vi "Microstrain IMU.vi"() -> ()   [LabVIEW 2012]
uses:
  <instrlib>/MicroStrain 3DM-GX1/MicroStrain 3DM-GX1.lvlib
  <vilib>/Platform/TimedLoop/XDataNode/wakeup.ctl
  <vilib>/Platform/TimedLoop/XDataNode/XDNodeRunTimeDep.lvlib
  <vilib>/Platform/TimedLoop/XDataNode/nitl_modes.ctl
  <vilib>/Platform/TimedLoop/XDataNode/timing_clust.ctl
  <vilib>/Platform/TimedLoop/XDataNode/XDataNode.xnode
  <vilib>/robotics/Controls/Compass Indicator/Compass Indicator.xctl
panel:
  out "VI Name":string
  out "Angle":dbl
  out "Waveform Chart 2":T1(graph)
  out "Waveform Chart":cluster{"Roll":dbl, "Pitch":dbl, "Yaw":dbl}(graph)
  in  "stop?":bool
  out "IMU Data":T2 {"Quaternion" format="%#.4g"; "Angular Rate"."Z-Axis Angular Rate" format="%#.4g"; "Angular Rate"."Y-Axis Angular Rate" format="%#.4g"; "Angular Rate"."X-Axis Angular Rate" format="%#.4g"; "Acceleration"."X-Axis Acceleration" format="%#.4g"; "Acceleration"."Y-Axis Acceleration" format="%#.4g"; "Acceleration"."Z-Axis Acceleration" format="%#.4g"; "Magnetic Field"."X-Axis Magnetic Field" format="%#.4g"; "Magnetic Field"."Y-Axis Magnetic Field" format="%#.4g"; "Magnetic Field"."Z-Axis Magnetic Field" format="%#.4g"; "Orientation Matrix" format="%#.4g"; "Position"."Yaw" format="%#.2f"; "Position"."Pitch" format="%#.1f"; "Position"."Roll" format="%#.1f"}
  in  "North Offset":dbl=30.0
  out "Compass Indicator":dbl(xcontrol)
  out "error out":errorcluster
  in  "Baud Rate":u32(ring)=115200 items=["19200"=19200, "38400"=38400, "115200"=115200]
  in  "Debug":bool
  in  "VISA resource name":refnum<visa-resource-name>="COM13"
  in  "Configure":bool
  out "Error Display":errorcluster
  in  "Enable Gyro-Stabilization (Enable)":bool=TRUE
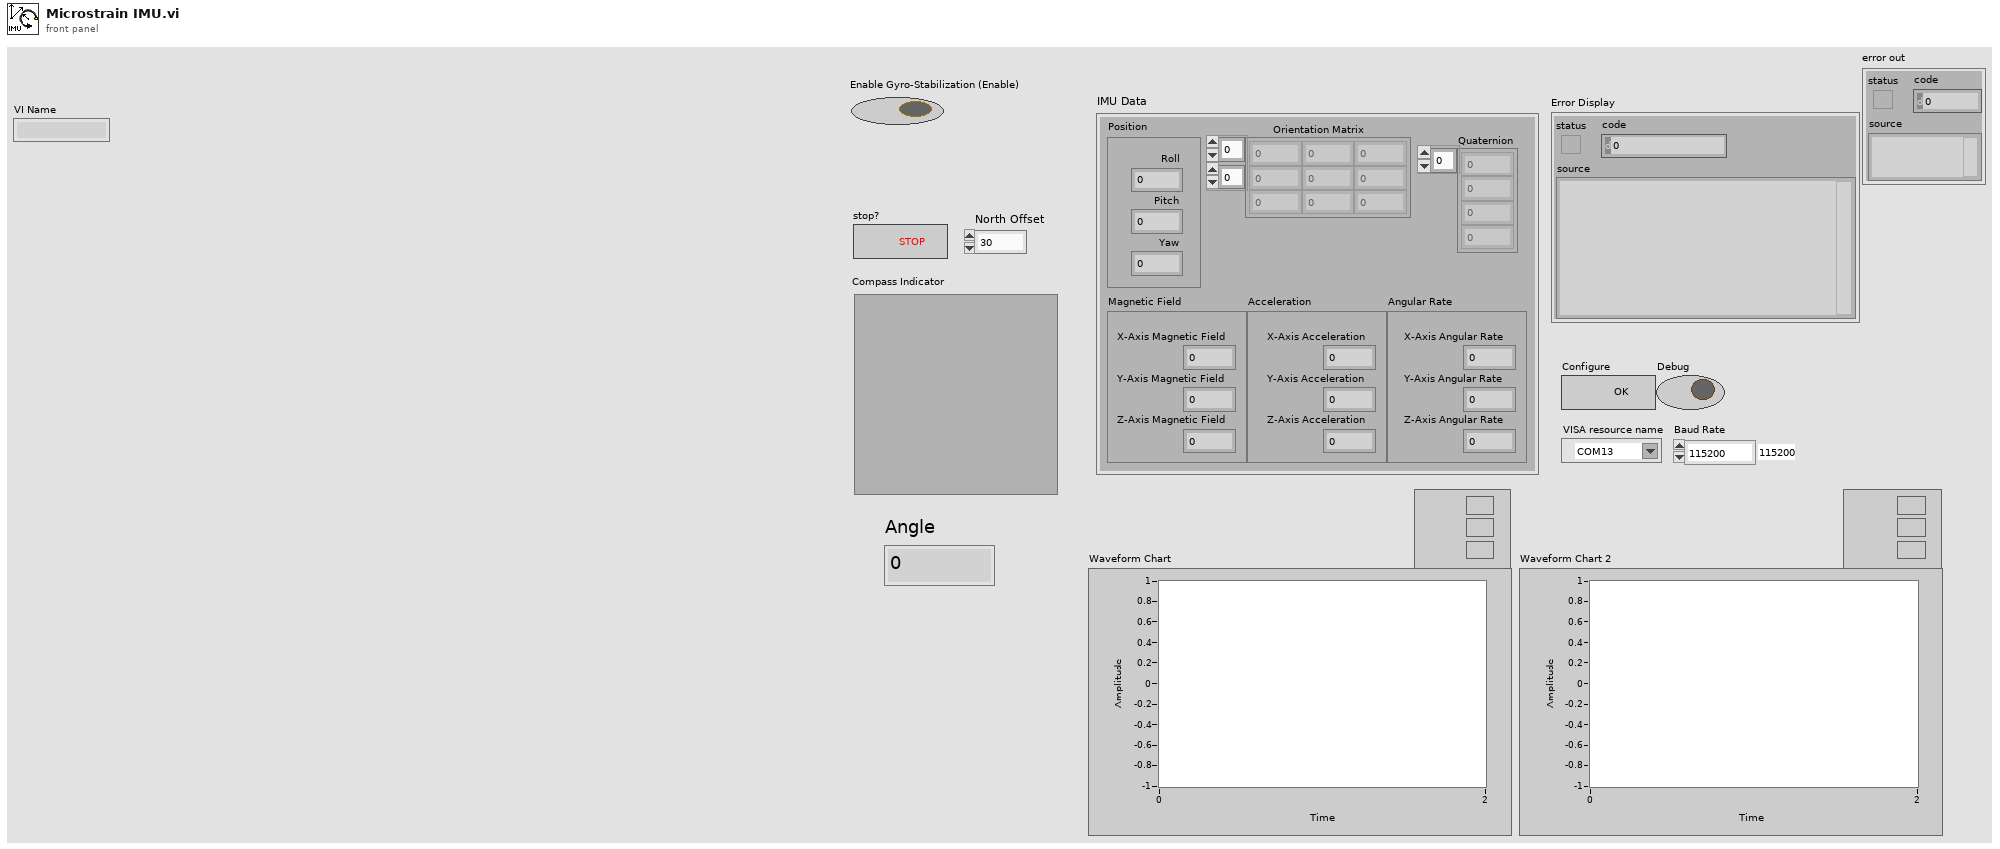
[diagram p1: front panel]
types:
  T1 = cluster{"X-Axis Magnetic Field":dbl, "Y-Axis Magnetic Field":dbl, "Z-Axis Magnetic Field":dbl}
  T2 = cluster{"Position":cluster{"Roll":dbl, "Pitch":dbl, "Yaw":dbl}, "Orientation Matrix":dbl[][], "Magnetic Field":cluster{"Z-Axis Magnetic Field":dbl, "Y-Axis Magnetic Field":dbl, "X-Axis Magnetic Field":dbl}, "Acceleration":cluster{"Z-Axis Acceleration":dbl, "Y-Axis Acceleration":dbl, "X-Axis Acceleration":dbl}, "Angular Rate":cluster{"X-Axis Angular Rate":dbl, "Y-Axis Angular Rate":dbl, "Z-Axis Angular Rate":dbl}, "Quaternion":dbl[]}
  T3 = typedef "XDNodeRunTimeDep.lvlib/timing_clust.ctl" = cluster{"Expected End [f-1]":u64, "Actual End [f-1]":u64, "Finished Late? [f-1]":bool, "Expected End [i-1]":u64, "Actual End [i-1]":u64, "Finished Late? [i-1]":bool, "Expected Start [i]":u64, "Actual Start [i]":u64, "Expected Start [f]":u64, "Actual Start [f]":u64, "Source Name":string, "Structure Name":string, "Period":i64, "Deadline":i64, "Offset":i64, "Start":i64, "Priority":i32, "Timeout":i32, "Mode":T4, "Wakeup Reason":T5, "Error":errorcluster, "Source Type":string, "Secondary Source Type":string, "Global End Time":u64, "Global Start Time":u64, "Frame Duration":u64, "Iteration Duration":u64, "Assigned CPU":i32, "I/O Scan Engine Mode":u32}
  T4 = typedef "XDNodeRunTimeDep.lvlib/nitl_modes.ctl" = enum32{"No Change", "Process missed periods, maintain original phase", "Discard missed periods, maintain original phase", "Process missed periods, ignore original phase", "Discard missed periods, ignore original phase"}
  T5 = typedef "XDNodeRunTimeDep.lvlib/wakeup.ctl" = enum32{"Normal", "Aborted", "Asynchronous wakeup", "Timing source error", "Timed loop error", "Timeout"}
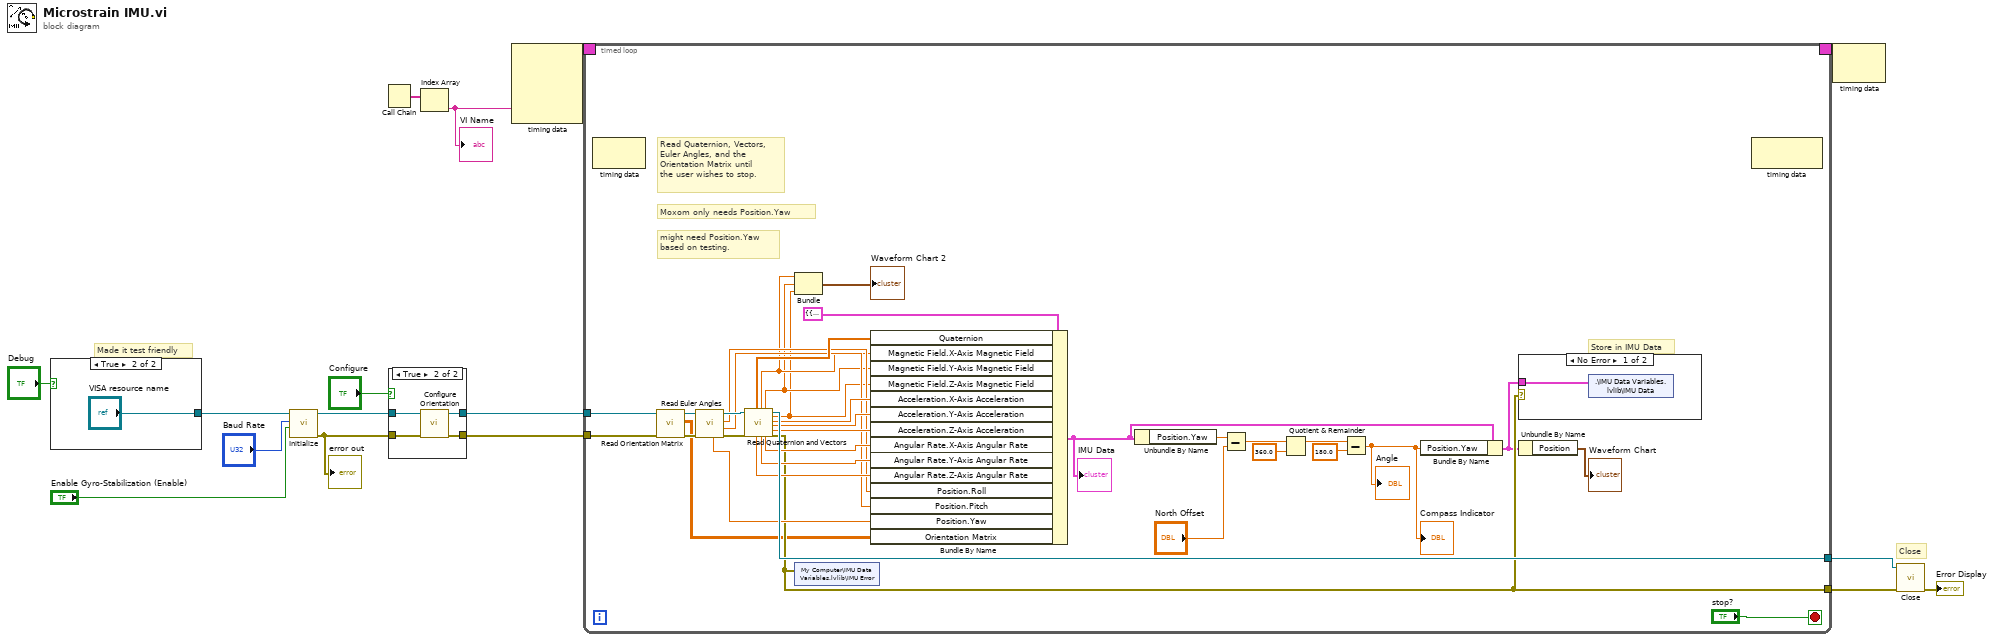
[diagram p0: block diagram]
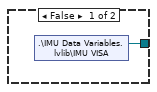
[diagram p3: hidden frame]
diagram:
  # "Made it test friendly"
  # "Close"
  n1 = case shown="True" "Debug" {
    tunnel: [w17 "VISA resource name"] -> w9
    frame False {
      n2 = shared-variable ".\\IMU Data Variables.lvlib\\IMU VISA"() -> (w17:refnum<visa-resource-name>)  [unwired: 1 in, 1 out]
    }
    frame True {
    }
  }
  n3 = call <instrlib>:"Initialize.vi"("Enable Gyro-Stabilization (True)"="Enable Gyro-Stabilization (Enable)", "Baud Rate (38400)"="Baud Rate", "VISA resource name"=w9) -> ("error out"=w13:errorcluster, "VISA resource name out"=w14:refnum<visa-resource-name>)  [unwired: 7 in]
  "error out" <- w13
  n4 = Call Chain() -> (call chain=w2:string[])
  n5 = case shown="True" "Configure" {
    tunnel: w14 -> [w20 w24]
    tunnel: w13 -> [w19 w23]
    tunnel: [w20 w22] -> w4
    tunnel: [w19 w21] -> w3
    frame False {
    }
    frame True {
      n6 = call <instrlib>:"Configure Orientation.vi"("error in (no error)"=w23, "VISA resource name"=w24) -> ("error out"=w21:errorcluster, "VISA resource name out"=w22:refnum<visa-resource-name>)  [unwired: 8 in]
    }
  }
  n7 = Index Array(array=w2) -> (element=w1:string)  [unwired: 1 in]
  "VI Name" <- w1
  n8 = node-c288(w1) -> (w16:T3)  [unwired: 3 in]
  n9 = timed-loop {
    tunnel: [w43] -> w12
    tunnel: [w57] -> w11
    timing: w16 -> [_]
    timing-out: [_] -> w15
    tunnel: w4 -> [w38]
    tunnel: w3 -> [w37]
    stop <- "stop?" stop-if-true
    # "Moxom only needs Position.Yaw"
    # "Store in IMU Data"
    # "might need Position.Yaw\nbased on testing."
    # "Read Quaternion, Vectors,\nEuler Angles, and the\nOrientation Matrix until\nthe user wishes to stop."
    n10 = node-c288() -> ()  [unwired: 1 in, 1 out]
    n11 = call <instrlib>:"Read Orientation Matrix.vi"("error in (no error)"=w37, "VISA resource name"=w38) -> ("error out"=w58:errorcluster, "Orientation Matrix"=w42:dbl[][], "VISA resource name out"=w59:refnum<visa-resource-name>)  [unwired: 7 in]
    n12 = call <instrlib>:"Read Euler Angles.vi"("error in (no error)"=w58, "VISA resource name"=w59) -> ("error out"=w55:errorcluster, "Pitch"=w44:dbl, "Roll"=w46:dbl, "VISA resource name out"=w56:refnum<visa-resource-name>, "Yaw"=w45:dbl)  [unwired: 5 in]
    n13 = call <instrlib>:"Read Quaternion and Vectors.vi"("VISA resource name"=w56, "error in (no error)"=w55) -> ("Quaternion"=w53:dbl[], "Z-Axis Angular Rate"=w47:dbl, "X-Axis Magnetic Field"=w36:dbl, "Y-Axis Angular Rate"=w48:dbl, "Y-Axis Magnetic Field"=w35:dbl, "X-Axis Angular Rate"=w49:dbl, "VISA resource name out"=w57:refnum<visa-resource-name>, "Z-Axis Magnetic Field"=w34:dbl, "X-Axis Acceleration"=w52:dbl, "Y-Axis Acceleration"=w51:dbl, "Z-Axis Acceleration"=w50:dbl, "error out"=w43:errorcluster)  [unwired: 6 in]
    n14 = Bundle("X-Axis Magnetic Field"=w36, "Y-Axis Magnetic Field"=w35, "Z-Axis Magnetic Field"=w34) -> (→"Waveform Chart 2":T1)  [unwired: 1 in]
    n15 = shared-variable "My Computer\\IMU Data Variables.lvlib\\IMU Error"(w43) -> ()  [unwired: 1 in, 1 out]
    n16 = Bundle By Name(cluster=T2 {"Position"={"Roll"=0.0, "Pitch"=0.0, "Yaw"=0.0}, "Orientation Matrix"=[], "Magnetic Field"={"Z-Axis Magnetic Field"=0.0, "Y-Axis Magnetic Field"=0.0, "X-Axis Magnetic Field"=0.0}, "Acceleration"={"Z-Axis Acceleration"=0.0, "Y-Axis Acceleration"=0.0, "X-Axis Acceleration"=0.0}, "Angular Rate"={"X-Axis Angular Rate"=0.0, "Y-Axis Angular Rate"=0.0, "Z-Axis Angular Rate"=0.0}, "Quaternion"=[]} ("IMU Data"), "Quaternion"=w53, "Magnetic Field.X-Axis Magnetic Field"=w36, "Magnetic Field.Y-Axis Magnetic Field"=w35, "Magnetic Field.Z-Axis Magnetic Field"=w34, "Acceleration.X-Axis Acceleration"=w52, "Acceleration.Y-Axis Acceleration"=w51, "Acceleration.Z-Axis Acceleration"=w50, "Angular Rate.X-Axis Angular Rate"=w49, "Angular Rate.Y-Axis Angular Rate"=w48, "Angular Rate.Z-Axis Angular Rate"=w47, "Position.Roll"=w46, "Position.Pitch"=w44, "Position.Yaw"=w45, "Orientation Matrix"=w42) -> (w41:T2)
    "IMU Data" <- w41
    n17 = Unbundle By Name(w41) -> ("Position.Yaw"=w40:dbl)
    n18 = Subtract(x=w40, y="North Offset") -> (x-y=w29:dbl)
    n19 = Quotient & Remainder(x=w29, y=360.0) -> (x-y*floor(x/y)=w28:dbl)  [unwired: 1 out]
    n20 = Subtract(x=w28, y=180.0) -> (x-y=w27:dbl)
    "Compass Indicator" <- w27
    "Angle" <- w27
    n21 = Bundle By Name(cluster=w41, "Position.Yaw"=w27) -> (w32:T2)
    n22 = case shown="No Error" w43 {
      tunnel: w32 -> [w62 _]
      frame No Error {
        n23 = shared-variable ".\\IMU Data Variables.lvlib\\IMU Data"(w62) -> ()  [unwired: 1 in, 1 out]
      }
      frame Error {
      }
    }
    n24 = Unbundle By Name(w32) -> ("Position"=→"Waveform Chart":cluster{"Roll":dbl, "Pitch":dbl, "Yaw":dbl})
    n25 = node-c288() -> ()  [unwired: 1 in, 1 out]
  }
  n26 = node-c288(w15) -> ()  [unwired: 1 out]
  n27 = call <instrlib>:"Close.vi"("error in (no error)"=w12, "VISA resource name"=w11) -> ("error out"=→"Error Display":errorcluster)  [unwired: 9 in]
